vi "DrawCursor.vi"(6 "Visible?":bool, 8 "error in (no error)":errorcluster, 11 "Highscore in":refnum<class "HighscoreDialog.lvclass">) -> (0 "error out":errorcluster, 3 "Highscore out":refnum<class "HighscoreDialog.lvclass">)   [LabVIEW 2019, in "RT_Game.lvlib" / "HighscoreDialog.lvclass"]
uses:
  HighscoreDialog.lvclass
  C:/Users/FreshBob/Dropbox/VIs/myRIO_GameConsole/RT/RT_Game/GameObject/GameObject.lvclass
  Engine/Coordinate.ctl
  GameObject/GameObject.lvclass/GameObject.ctl
  HighscoreDialog.lvclass/HighscoreDialog.ctl
  GameObject/Read position.vi
  Engine/Engine.lvclass
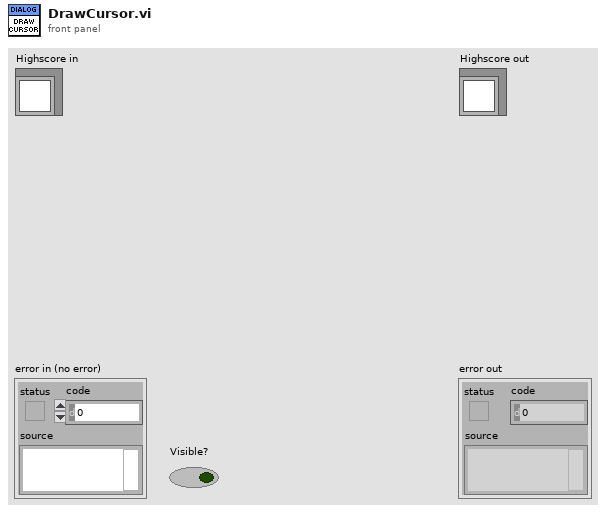
[diagram p1: front panel]
types:
  T1 = typedef "RT_Game.lvlib/Engine.lvclass/Coordinate.ctl" = cluster{"x":dbl, "y":dbl}
  T2 = typedef "RT_Game.lvlib/Game.lvclass/Coordinate.ctl" = cluster{"x":dbl, "y":dbl}
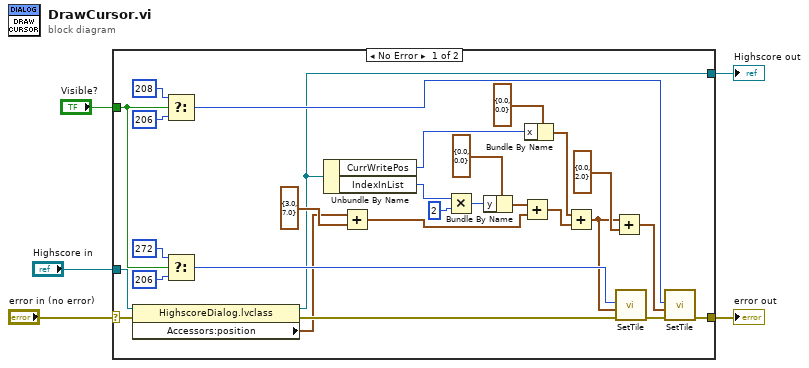
[diagram p0: block diagram]
diagram:
  n1 = case shown="No Error" "error in (no error)" {
    selector: "error in (no error)" -> [w33 w35]
    tunnel: [w31 w35] -> w4
    tunnel: [w8 w34] -> w2
    tunnel: "Highscore in" -> [w9 w34]
    tunnel: "Visible?" -> [w24 _]
    frame No Error {
      n2 = property class="HighscoreDialog.lvclass"(reference=w9, error in=w33) -> (reference out=w8:refnum<class "HighscoreDialog.lvclass">, error out=w10:errorcluster, "Accessors:position"=w7:T2)
      n3 = Select(t=u32 208 ("TileNumber"), s=w24, f=u32 206) -> (s? t:f=w25:u32)
      n4 = Select(t=u32 272 ("TileNumber"), s=w24, f=u32 206) -> (s? t:f=w29:u32)
      n5 = Unbundle By Name(w8) -> ("CurrWritePos"=w13:i16, "IndexInList"=w6:i16)
      n6 = Add(x=w7, y=T1 {"x"=3.0, "y"=7.0}) -> (x+y=w21:T2)
      n7 = Multiply(x=w6, y=i16 2) -> (x*y=w18:i16)
      n8 = Bundle By Name(cluster=T1 {"x"=0.0, "y"=0.0} ("x"), "y"=w18) -> (w19:T1)
      n9 = Add(x=w19, y=w21) -> (x+y=w11:T1)
      n10 = Bundle By Name(cluster=T1 {"x"=0.0, "y"=0.0} ("x"), "x"=w13) -> (w14:T1)
      n11 = Add(x=w14, y=w11) -> (x+y=w12:T1)
      n12 = Add(x=w12, y=T1 {"x"=0.0, "y"=2.0}) -> (x+y=w16:T1)
      n13 = call "SetTile.vi"("error in (no error)"=w10, "Coordinates"=w12, "TileCode"=w29) -> ("error out"=w32:errorcluster)  [unwired: 8 in]
      n14 = call "SetTile.vi"("error in (no error)"=w32, "Coordinates"=w16, "TileCode"=w25) -> ("error out"=w31:errorcluster)  [unwired: 8 in]
    }
    frame Error {
    }
  }
  "error out" <- w4
  "Highscore out" <- w2
